vi "PackConvertModule.vi"(6 "3 in":u8, 7 "4":u8, 9 "2 in":u8, 10 "1 in":u8, 11 "0 in":u8) -> (1 "2 out":u16, 2 "1 out":u16, 3 "0 out":u16, 4 "3 out":u16)   [LabVIEW 2013]
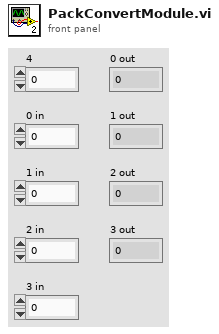
[diagram p1: front panel]
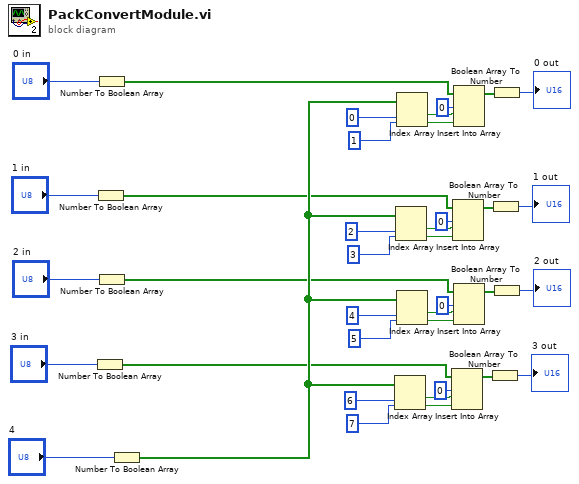
[diagram p0: block diagram]
diagram:
  n1 = Number To Boolean Array(number="3 in") -> (Boolean array=w35:bool[])
  n2 = Number To Boolean Array(number="1 in") -> (Boolean array=w17:bool[])
  n3 = Number To Boolean Array(number="0 in") -> (Boolean array=w8:bool[])
  n4 = Number To Boolean Array(number="2 in") -> (Boolean array=w26:bool[])
  n5 = Number To Boolean Array(number="4") -> (Boolean array=w38:bool[])
  n6 = Index Array(array=w38, index #1=6 ("index"), index #2=7 ("index")) -> (element #1=w30:bool, element #2=w31:bool)
  n7 = Index Array(array=w38, index #1=2 ("index"), index #2=3 ("index")) -> (element #1=w12:bool, element #2=w13:bool)
  n8 = Index Array(array=w38, index #1=0 ("index"), index #2=1 ("index")) -> (element #1=w3:bool, element #2=w4:bool)
  n9 = Index Array(array=w38, index #1=4 ("index"), index #2=5 ("index")) -> (element #1=w21:bool, element #2=w22:bool)
  n10 = Insert Into Array(array=w35, index=0, new element #1=w30, new element #2=w31) -> (w36:bool[])
  n11 = Insert Into Array(array=w17, index=0, new element #1=w12, new element #2=w13) -> (w18:bool[])
  n12 = Insert Into Array(array=w8, index=0, new element #1=w3, new element #2=w4) -> (w9:bool[])
  n13 = Insert Into Array(array=w26, index=0, new element #1=w21, new element #2=w22) -> (w27:bool[])
  n14 = Boolean Array To Number(Boolean array=w36) -> (number=→"3 out":u32)
  n15 = Boolean Array To Number(Boolean array=w18) -> (number=→"1 out":u32)
  n16 = Boolean Array To Number(Boolean array=w9) -> (number=→"0 out":u32)
  n17 = Boolean Array To Number(Boolean array=w27) -> (number=→"2 out":u32)
